vi "FTW-Endpoint-Pipe-Connect.vi"(0 "FTW Endpoint":refnum<class "FTW-Endpoint.lvclass">, 11 "error in":errorcluster) -> (4 "FTW Endpoint out":refnum<class "FTW-Endpoint.lvclass">, 15 "error out":errorcluster)   [LabVIEW 2013, in "FTW-Endpoint.lvclass"]
doc: "Connect the base endpoint to its own pipe, primarily for reply purposes."
uses:
  FTW-Endpoint.lvclass
  FTW-Endpoint.lvclass/FTW-Endpoint.ctl
panel:
  # "Inputs"
  # "Outputs"
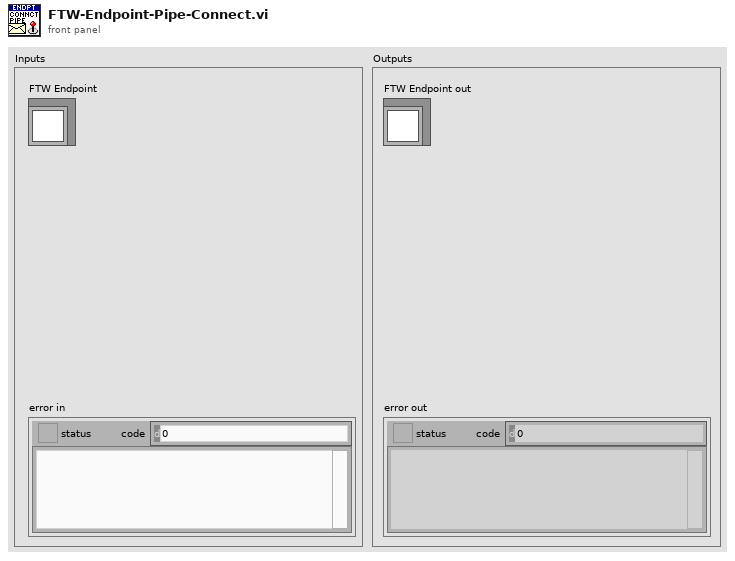
[diagram p1: front panel]
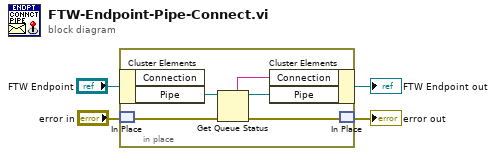
[diagram p0: block diagram]
diagram:
  n1 = in-place {
    n2 = in-place-cluster #1("FTW Endpoint") -> ("Pipe"=w7:refnum<queue>)  [unwired: 1 out]
    n3 = in-place-match #2("error in") -> (w5:errorcluster)
    n4 = Get Queue Status(queue=w7, error in (no error)=w5) -> (queue out=w9:refnum<queue>, queue name=w6:string, error out=w8:errorcluster)  [unwired: 1 in, 5 out]
    n5 = in-place-cluster #1("Connection"=w6, "Pipe"=w9) -> (→"FTW Endpoint out":refnum<class "FTW-Endpoint.lvclass">)
    n6 = in-place-match #2(w8) -> (→"error out":errorcluster)
  }
